vi "Initialise Data Bus Task.vi"(8 "error in":errorcluster) -> (0 "error out":errorcluster, 3 "Data Bus":refnum<k21> caption="task out")   [LabVIEW 2021, in "IO.lvclass"]
uses:
  IO.lvclass
  <vilib>/DAQmx/create/channels.llb/DAQmx Create Channel (DO-Digital Output).vi
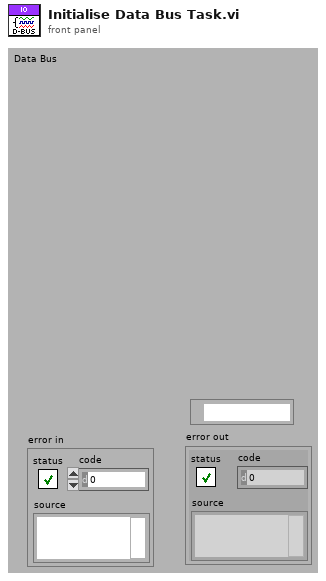
[diagram p1: front panel]
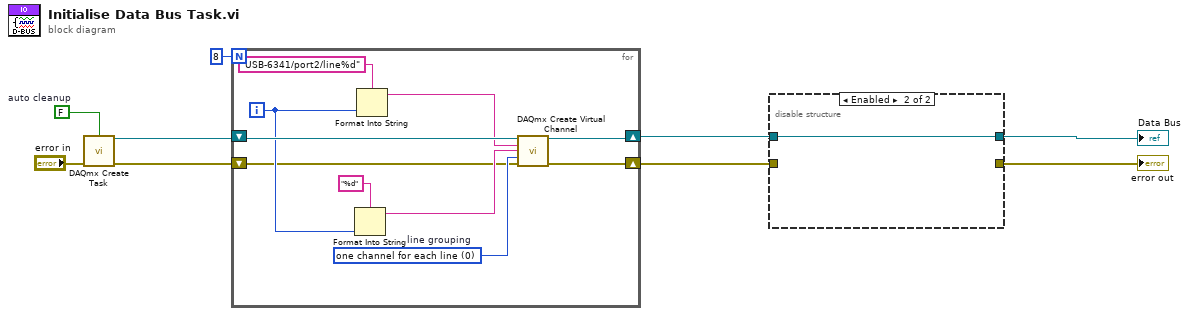
[diagram p0: block diagram]
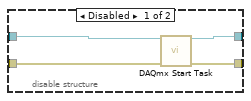
[diagram p2: hidden frame]
diagram:
  w8 = FALSE  # auto cleanup
  n1 = call <vilib>:"DAQmx Create Task.vi"("auto cleanup"=w8, "error in"="error in") -> ("task out"=w4:refnum<k21>, "error out"=w5:errorcluster)  [unwired: 12 in]
  n2 = for {
    N: 8 -> [_]
    shift-right: [w18] -> w3
    shift-left: w4 -> [w17]
    shift-right: [w11] -> w2
    shift-left: w5 -> [w10]
    i -> [w12]
    w19 = 0 items=["one channel for each line", "one channel for all lines"]  # line grouping
    n3 = Format Into String(format string="%d" ("lines"), w12) -> (resulting string=w13:string)  [unwired: 2 in, 1 out]
    n4 = Format Into String(format string="USB-6341/port2/line%d" ("lines"), w12) -> (resulting string=w15:string)  [unwired: 2 in, 1 out]
    n5 = call-poly <vilib>:"DAQmx Create Virtual Channel.vi"("task in"=w17, "lines"=w15, "name to assign"=w13, "line grouping"=w19, "error in"=w10) -> ("task out"=w18:refnum<k21>, "error out"=w11:errorcluster)  [unwired: 9 in]
  }
  n6 = disable-structure shown="Enabled" {
    disable-tunnel: w3 -> [w23 w24]
    disable-tunnel: [w22 w24] -> w7
    disable-tunnel: w2 -> [w21 _]
    disable-tunnel: [w20 _] -> w6
    frame Disabled {
      n7 = call <vilib>:"DAQmx Start Task.vi"("task/channels in"=w23, "error in"=w21) -> ("task out"=w22:refnum<k21>, "error out"=w20:errorcluster)  [unwired: 12 in]
    }
    frame Enabled {
    }
  }
  "error out" <- w6
  "Data Bus" <- w7
